vi "Write Variant.vi"(8 "error in (no error)":errorcluster, 10 "Variant":variant, 11 "JSONPacket in":refnum<class "JSONPacket.lvclass">) -> (0 "error out":errorcluster, 3 "JSONPacket out":refnum<class "JSONPacket.lvclass">)   [LabVIEW 2019]
uses:
  JSONPacket.lvclass
  C:/projects/labview_multiplayer_snake_personal/Main Codeline/Software/Code/Shared/TCPPacket/TCPPacket.lvclass
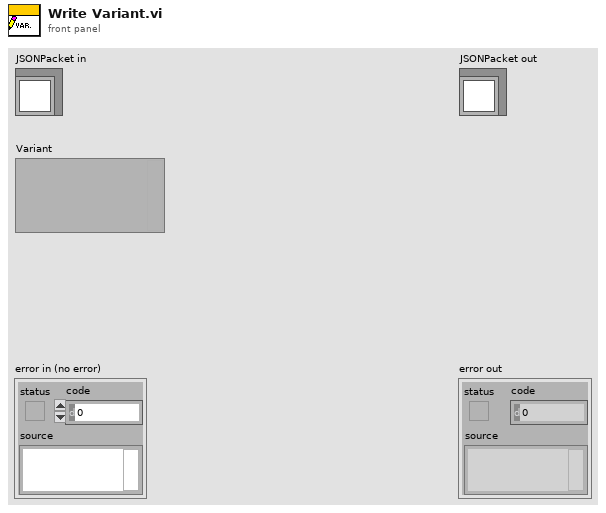
[diagram p1: front panel]
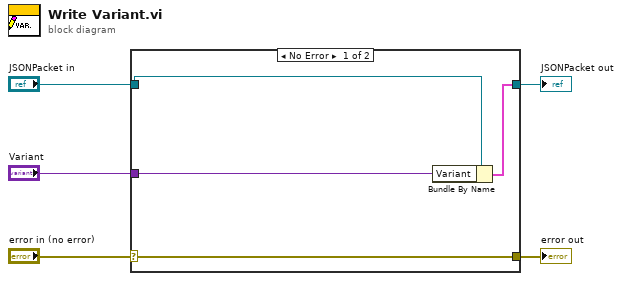
[diagram p0: block diagram]
diagram:
  n1 = case shown="No Error" "error in (no error)" {
    selector: "error in (no error)" -> [w9 w10]
    tunnel: [w9 w10] -> w4
    tunnel: [w7 w11] -> w2
    tunnel: "JSONPacket in" -> [w8 w11]
    tunnel: "Variant" -> [w6 _]
    frame No Error {
      n2 = Bundle By Name(cluster=w8, "Variant"=w6) -> (w7:cluster{})
    }
    frame Error {
    }
  }
  "error out" <- w4
  "JSONPacket out" <- w2
